vi "configure enable channel.vi"(8 "error in":errorcluster, 10 "tag in":string, 11 "node in":refnum<data-value>) -> (0 "error out":errorcluster, 1 "success":bool, 2 "tag out":string, 3 "node out":refnum<data-value>, 5 "changed":bool)   [LabVIEW 2013, in "TDMS datalogger editor node.lvclass"]
uses:
  TDMS datalogger editor node.lvclass
  <vilib>/CEF_TreeControl/Node/NISE_CEF_Node.lvclass
  <vilib>/NI/Tag Bus/tag/Data Type.ctl
  <vilib>/NI/Tag Bus/tag/tag descriptor.lvclass
  <vilib>/NI/Component Execution Engine/Configuration Editor/Classes/EngineTags/EngineTags.lvclass
panel:
  in  "Linked Tag":u16(ring) items=["", "testbool"]
  in  "cancel":bool
  in  "ok":bool
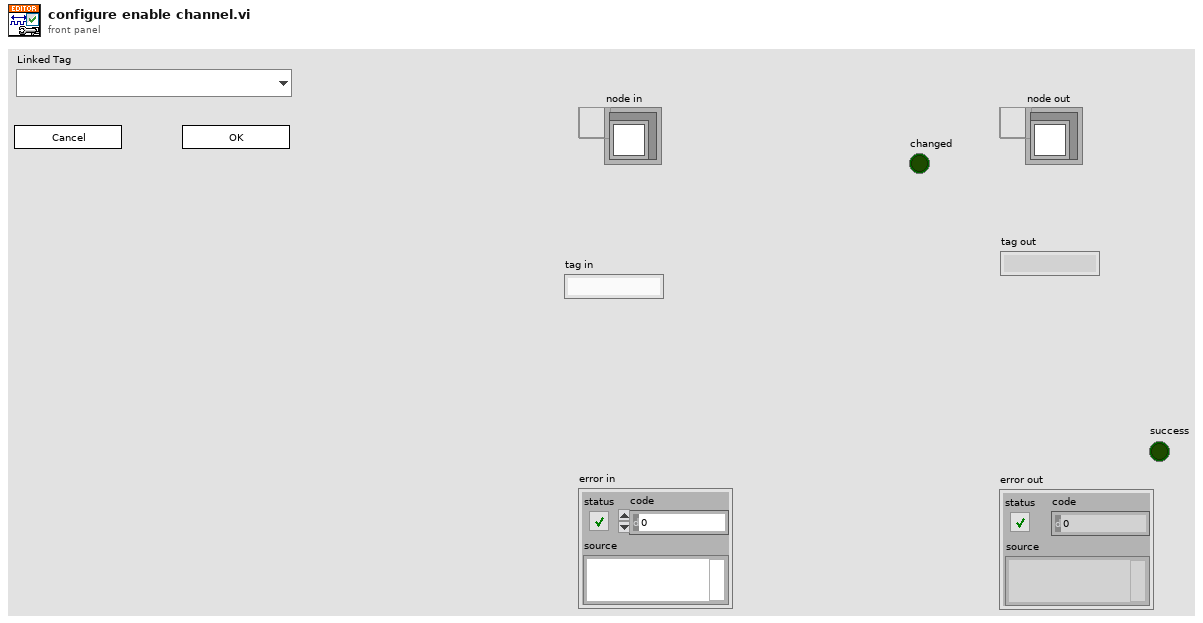
[diagram p1: front panel]
types:
  T1 = typedef "tag bus.lvlib/tag descriptor.lvclass/Data Type.ctl" = enum16{"Double", "Single", "I64", "I32", "I16", "I8", "U64", "U32", "U16", "U8", "Boolean", "String", "Array of Double", "Array of Single", "Array of I64", "Array of I32", "Array of I16", "Array of I8", "Array of U64", "Array of U32", "Array of U16", "Array of U8", "Array of Boolean", "Array of String"}
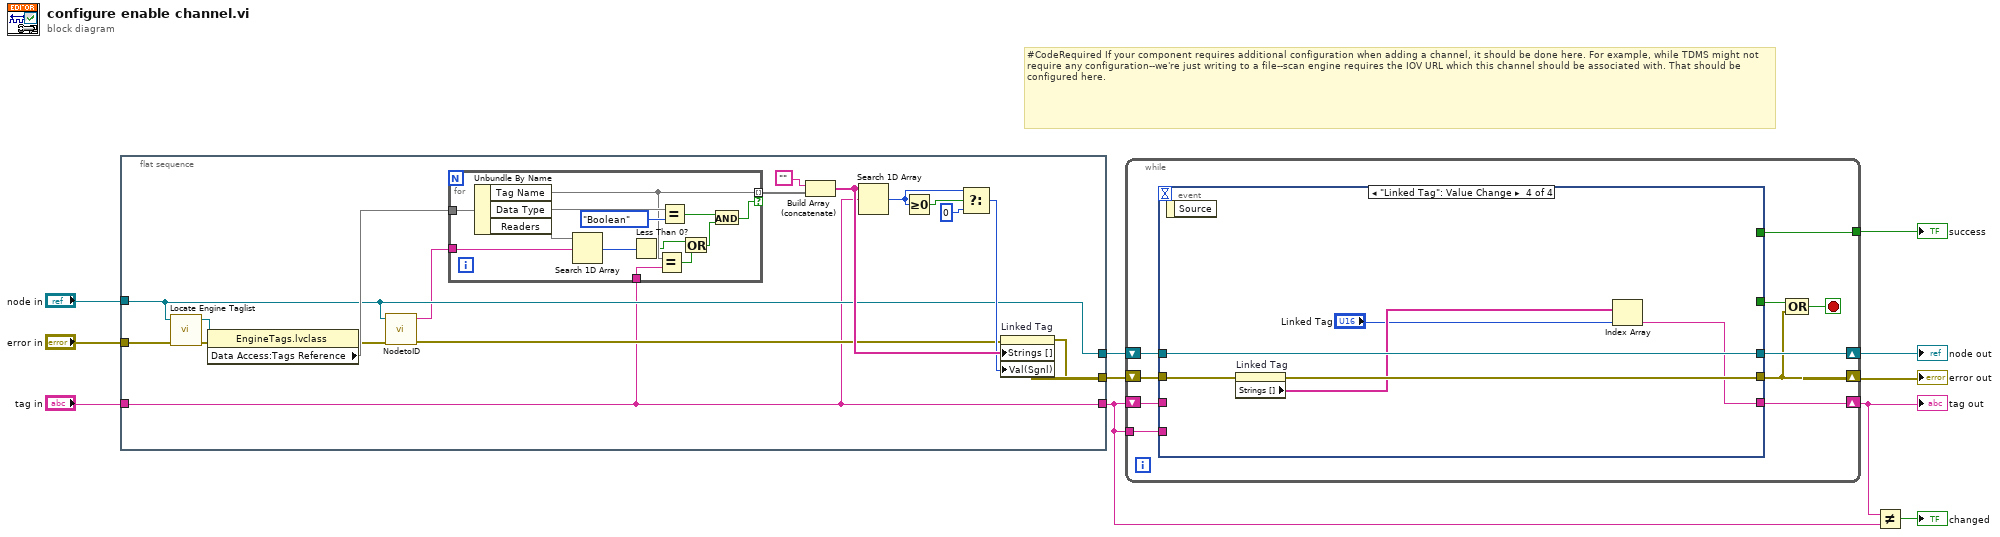
[diagram p0: block diagram]
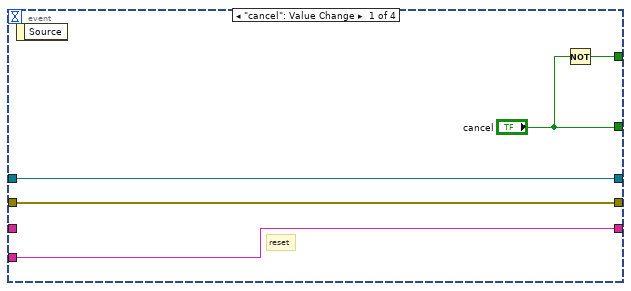
[diagram p2: hidden frame]
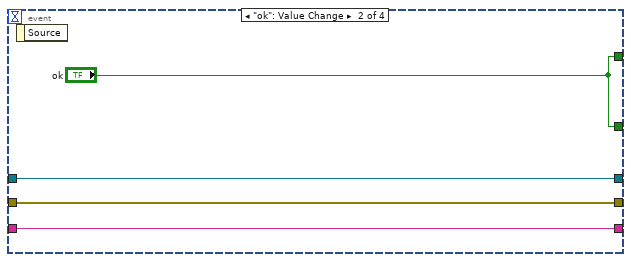
[diagram p3: hidden frame]
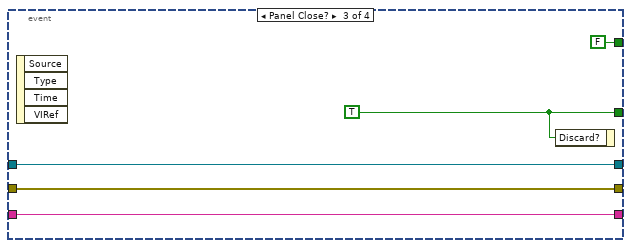
[diagram p4: hidden frame]
diagram:
  # "#CodeRequired If your component requires additional configuration when adding a channel, it should be done here. For example, while TDMS might not require any configuration--we're just writing to a file--scan engine requires the IOV URL which this channel should be associated with. That should be configured here."
  n1 = flat-sequence {
    tunnel: [w28] -> w9
    tunnel: "error in" -> [w19]
    tunnel: [w15] -> w10
    tunnel: "tag in" -> [w12]
    tunnel: [w12] -> w2
    tunnel: "node in" -> [w15]
    frame #0 {
      n2 = call <vilib>:"Locate Engine Taglist.vi"("error in"=w19, "node ref"=w15) -> ("error out"=w26:errorcluster, "EngineTags"=w27:refnum<data-value>)  [unwired: 8 in]
      n3 = property class="EngineTags.lvclass"(reference=w27, error in=w26) -> (error out=w17:errorcluster, "Data Access:Tags Reference"=w18)  [unwired: 1 out]
      n4 = call <vilib>:"NodetoID.vi"("error in"=w17, "node ref"=w15) -> ("error out"=w16:errorcluster, "ID"=w14:string)  [unwired: 8 in]
      n5 = for {
        tunnel: w18 -> [w41]
        tunnel: w14 -> [w36]
        tunnel: [w30] -> w13 mode=indexing if=w34
        tunnel: w12 -> [w33]
        n6 = Unbundle By Name(w41) -> ("Tag Name"=w30, "Data Type"=w40, "Readers"=w37)
        n7 = Search 1D Array(1D array=w37, element=w36) -> (index of element=w35:i32)  [unwired: 1 in]
        n8 = Less Than 0?(x=w35) -> (x < 0?=w29:bool)
        n9 = Equal?(x=w30, y=w33) -> (x = y?=w31:bool)
        n10 = Equal?(x=w40, y=Data_Type."Boolean") -> (x = y?=w38:bool)
        n11 = Or(x=w29, y=w31) -> (x .or. y?=w32:bool)
        n12 = And(x=w38, y=w32) -> (x .and. y?=w34:bool)
      }
      n13 = Build Array (concatenate)("", w13) -> (w21:string[])
      n14 = Search 1D Array(1D array=w21, element=w12) -> (index of element=w24:i32)  [unwired: 1 in]
      n15 = Greater Or Equal To 0?(x=w24) -> (x >= 0?=w23:bool)
      n16 = Select(t=w24, s=w23, f=0) -> (s? t:f=w20:i32)
      n17 = property on="Linked Tag" class="Ring (strict)"(error in=w16, "Strings []"=w21, "Val(Sgnl)"=w20) -> (error out=w28:errorcluster)  [unwired: 1 in, 1 out]
    }
  }
  n18 = while {
    shift-right: [w46] -> w6
    shift-left: w9 -> [w50]
    shift-right: [w49] -> w7
    shift-left: w10 -> [w51]
    tunnel: [w48] -> w8
    shift-right: [w43] -> w5
    shift-left: w2 -> [w44]
    tunnel: w2 -> [w42]
    stop <- w45 stop-if-true
    n19 = event shown="[3] \"Linked Tag\": Value Change" {
      selector: _ -> [_ _ _ _]
      dyn-events: _ -> [_ _ _ _]
      timeout: _ -> [_ _ _ _]
      tunnel: w51 -> [w56 w60 w65 w71]
      tunnel: w50 -> [w55 w58 w64 w70]
      tunnel: [w56 w60 w65 w71] -> w49
      tunnel: [w55 w58 w64 w69] -> w46
      tunnel: [w54 "ok" FALSE _] -> w48
      tunnel: ["cancel" "ok" w62 _] -> w47
      tunnel: w44 -> [_ w59 w61 _]
      tunnel: [w52 w59 w61 w66] -> w43
      tunnel: w42 -> [w52 _ _ _]
      event "cancel": Value Change {
        # "reset"
        n20 = event-data() -> ()  [unwired: 1 in, 1 out]
        n21 = Not(x="cancel") -> (.not. x?=w54:bool)
      }
      event "ok": Value Change {
        n22 = event-data() -> ()  [unwired: 1 in, 1 out]
      }
      event Panel Close? {
        w62 = TRUE ("cancel")
        n23 = event-data() -> ()  [unwired: 1 in, 4 out]
        n24 = event-data("Discard?"=w62) -> ()  [unwired: 1 in, 1 out]
      }
      event "Linked Tag": Value Change {
        n25 = event-data() -> ()  [unwired: 1 in, 1 out]
        n26 = property on="Linked Tag" class="Ring (strict)"(error in=w70) -> (error out=w69:errorcluster, "Strings []"=w68:string[])  [unwired: 1 in, 1 out]
        n27 = Index Array(array=w68, index="Linked Tag") -> (element=w66:string)
      }
    }
    n28 = Compound Arithmetic op=OR(w47, w46) -> (w45:bool)
  }
  "error out" <- w6
  "success" <- w8
  "node out" <- w7
  "tag out" <- w5
  n29 = Not Equal?(x=w5, y=w2) -> (x != y?=→"changed":bool)
